vi "Control Value Update (Boolean).vi"(0 "Software Value":bool, 5 "Hardware Value":bool) -> (14 "New Software Value":bool, 15 "Update Software":bool, 18 "New Hardware Value":bool, 19 "Update Hardware":bool)   [LabVIEW 2011]
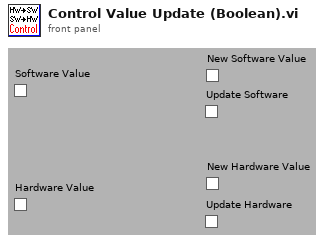
[diagram p1: front panel]
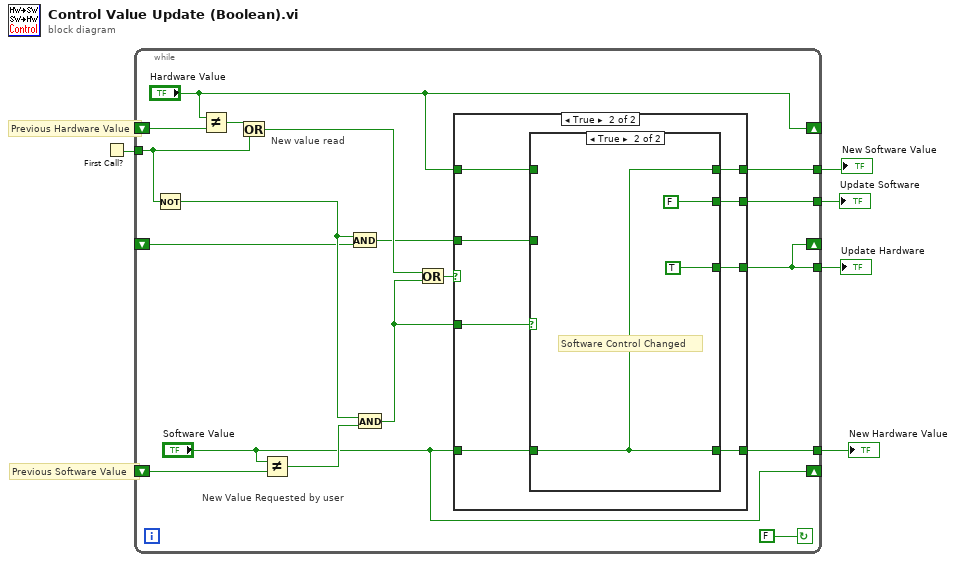
[diagram p0: block diagram]
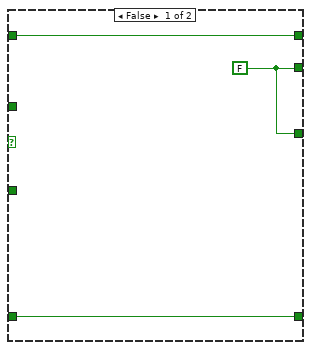
[diagram p2: hidden frame]
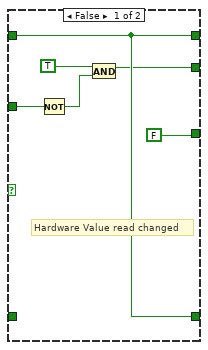
[diagram p3: hidden frame]
diagram:
  # "Previous Software Value"
  # "Previous Hardware Value"
  n1 = First Call?() -> (First Call?: T/F=w3:bool)
  n2 = while {
    tunnel: w3 -> [w22]
    shift-left: _ -> [w20]
    shift-right: ["Hardware Value"] -> _
    shift-right: ["Software Value"] -> _
    shift-left: _ -> [w19]
    tunnel: [w17] -> w5
    tunnel: [w13] -> w4
    shift-right: [w13] -> _
    shift-left: _ -> [w11]
    tunnel: [w9] -> w2
    tunnel: [w8] -> w1
    stop <- FALSE continue-if-true
    # "New Value Requested by user"
    # "New value read"
    n3 = Not(x=w22) -> (.not. x?=w12:bool)
    n4 = Not Equal?(x="Hardware Value", y=w20) -> (x != y?=w23:bool)
    n5 = Or(x=w23, y=w22) -> (x .or. y?=w14:bool)
    n6 = Not Equal?(x="Software Value", y=w19) -> (x != y?=w21:bool)
    n7 = And(x=w12, y=w11) -> (x .and. y?=w10:bool)
    n8 = And(x=w12, y=w21) -> (x .and. y?=w15:bool)
    n9 = Or(x=w14, y=w15) -> (x .or. y?=w18:bool)
    n10 = case shown="True" w18 {
      tunnel: "Hardware Value" -> [w26 w34]
      tunnel: [w25 w33] -> w17
      tunnel: [w25 w32] -> w13
      tunnel: [w26 w31] -> w9
      tunnel: [w24 w30] -> w8
      tunnel: "Software Value" -> [w24 w29]
      tunnel: w15 -> [_ w28]
      tunnel: w10 -> [_ w27]
      frame False {
        w25 = FALSE
      }
      frame True {
        n11 = case shown="True" w28 {
          tunnel: w34 -> [w40 _]
          tunnel: [w35 FALSE] -> w33
          tunnel: [FALSE TRUE] -> w32
          tunnel: [w40 w42] -> w31
          tunnel: [w40 w42] -> w30
          tunnel: w29 -> [_ w42]
          tunnel: w27 -> [w38 _]
          frame False {
            # "Hardware Value read changed"
            n12 = Not(x=w38) -> (.not. x?=w36:bool)
            n13 = And(x=TRUE, y=w36) -> (x .and. y?=w35:bool)
          }
          frame True {
            # "Software Control Changed"
          }
        }
      }
    }
  }
  "New Software Value" <- w2
  "Update Software" <- w5
  "Update Hardware" <- w4
  "New Hardware Value" <- w1
